vi "WSVCAP SHL FPGA LL Procedure I2C - Read ACK.vi"(0 "Procedure Step":T1, 1 "Wait Ticks Remaining":u32, 7 "I2C Wait Ticks":u32, 9 "Socket Mask":u64 format="%012x", 11 "error in (no error)":errorcluster, 14 "UUT Set (0/1)":u8) -> (3 "Wait Ticks Remaining Out":u32, 4 "Procedure Step Out":T1, 8 "Finished":bool, 10 "ACK Bit Read":u64, 15 "error out":errorcluster)   [LabVIEW 2017]
uses:
  Type Defs/WSVCAP SHL Procedure Step Enum.ctl
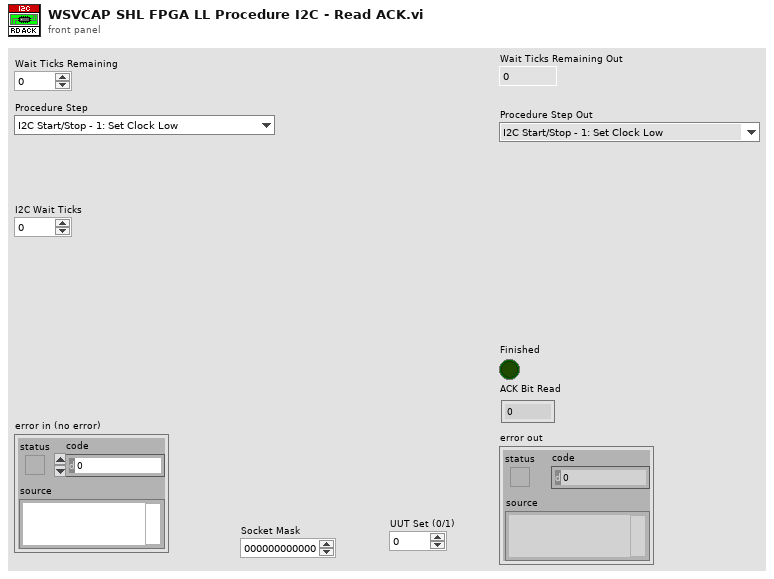
[diagram p1: front panel]
types:
  T1 = typedef "WSVCAP SHL Procedure Step Enum.ctl" = enum16{"I2C Start/Stop - 1: Set Clock Low", "I2C Start/Stop - 2: Wait", "I2C Start/Stop - 3: Set Data I", "I2C Start/Stop - 4: Wait", "I2C Start/Stop - 5: Set Clock High", "I2C Start/Stop - 6: Wait", "I2C Start/Stop - 7: Set Data II", "I2C Start/Stop - 8: Wait", "I2C Start/Stop - 9: Set Clock Low", "I2C Start/Stop - 10: Wait", "I2C Read ACK - 1: Set Clock High", "I2C Read ACK - 2: Wait", "I2C Read ACK - 3: Read ACK Bit", "I2C Read ACK - 4: Wait", "I2C Read ACK - 5: Set Clock Low", "I2C Read ACK - 6: Wait", "I2C Write ACK - 1: Write ACK Bit", "I2C Write ACK - 2: Wait", "I2C Write ACK - 3: Set Clock High", "I2C Write ACK - 4: Wait", "I2C Write ACK - 5: Set Clock Low", "I2C Write ACK - 6: Wait", "I2C Write ACK - 7: Set Data Low", "I2C Send Add - 1: Reset Bits Remaining", "I2C Send Add - 2: Set Data Bit", "I2C Send Add - 3: Wait", "I2C Send Add - 4: Set Clock High", "I2C Send Add - 5: Wait", "I2C Send Add - 6: Set Clock Low", "I2C Send Add - 7: Wait", "I2C Send Add - 8: Check Bits Remaining", "I2C Send Data - 1: Reset Bits Remaining", "I2C Send Data - 2: Load Write Bit from FIFO", "I2C Send Data - 3: Set Data Bit", "I2C Send Data - 4: Wait", "I2C Send Data - 5: Set Clock High", "I2C Send Data - 6: Wait", "I2C Send Data - 7: Set Clock Low", "I2C Send Data - 8: Wait", "I2C Send Data - 9: Check Bits Remaining", "I2C Receive Data - 1: Reset Bits Remaining", "I2C Receive Data - 2: Wait", "I2C Receive Data - 3: Set Clock High", "I2C Receive Data - 4: Wait", "I2C Receive Data - 5: Read Data Bit", "I2C Receive Data - 6: Wait", "I2C Receive Data - 7: Set Clock Low", "I2C Receive Data - 8: Wait", "I2C Receive Data - 9: Check Bits Remaining", "RFFE Send SSC - 1:Set Low", "RFFE Send SSC - 2:Wait", "RFFE Send SSC - 3:Set SDA High", "RFFE Send SSC - 4:Wait", "RFFE Send SSC - 5:Set SDA Low", "RFFE Send SSC - 6:Wait", "RFFE Send Data - 1:Set SCL High", "RFFE Send Data - 2:Wait", "RFFE Send Data - 3:Set SCL Low", "RFFE Send Data - 4:Wait", "RFFE Send Data - 5:Set SCL High (P)", "RFFE Send Data - 6:Wait", "RFFE Send Data - 7:Set SCL Low (P)", "RFFE Send Data - 8:Wait", "RFFE Send Data - 9:Set SCL High (BP)", "RFFE Send Data - 10:Wait", "RFFE Send Data - 11:Set SCL Low (BP)", "RFFE Send Data - 12:Wait", "RFFE Receive Data - 1:Set SCL High", "RFFE Receive Data - 2:Wait", "RFFE Receive Data - 3:Set SCL Low", "RFFE Receive Data - 4:Wait", "RFFE Receive Data - 5:Set SCL High (BP)", "RFFE Receive Data - 6:Wait", "RFFE Receive Data - 7:Set SCL Low (BP)", "RFFE Receive Data - 8:Wait", "RFFE Wait CMD Delay - 1:Wait", "RFFE Clear Lines - 1:Clear"}
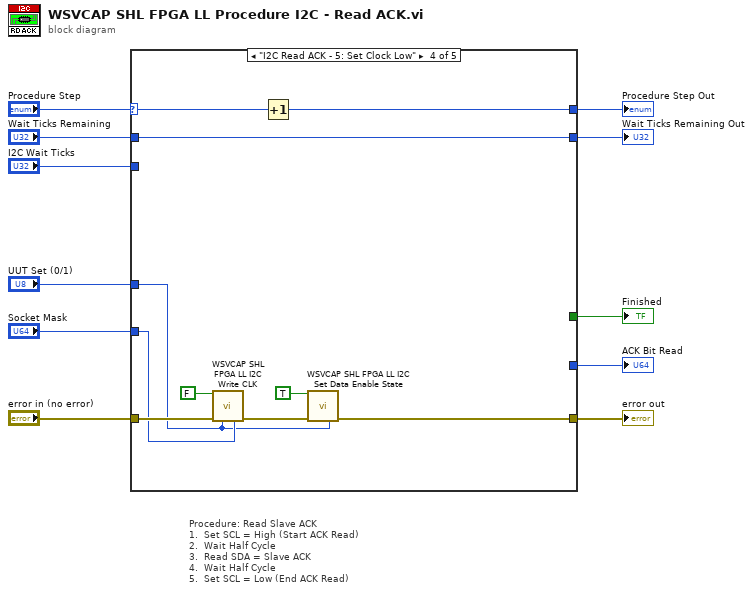
[diagram p0: block diagram]
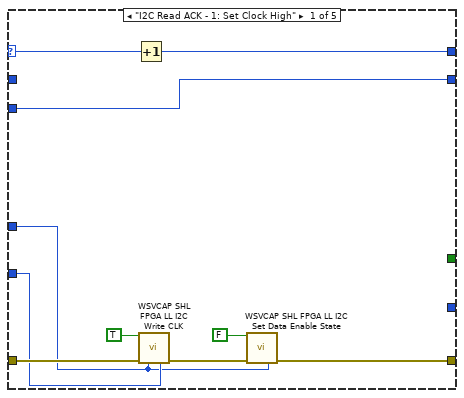
[diagram p2: hidden frame]
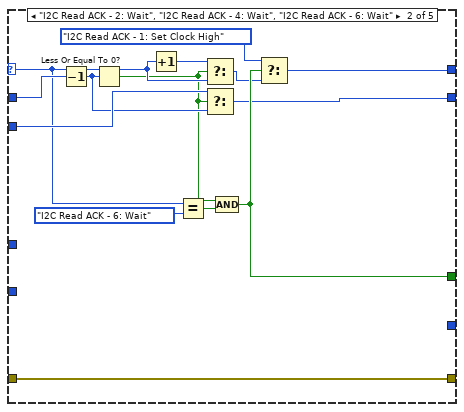
[diagram p3: hidden frame]
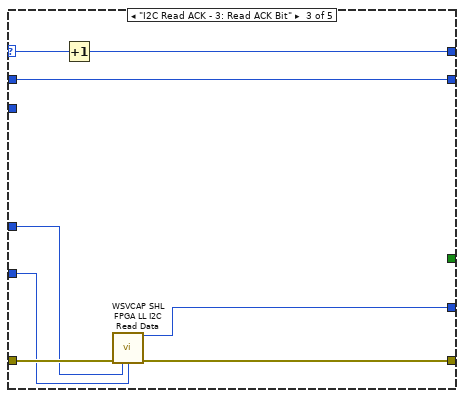
[diagram p4: hidden frame]
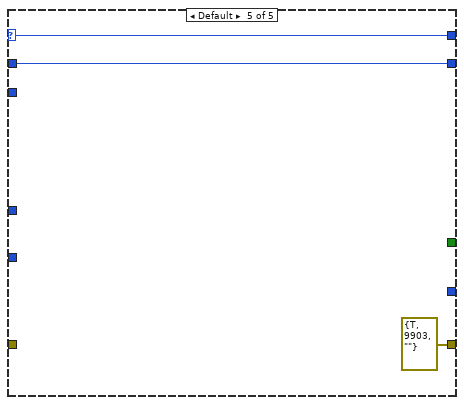
[diagram p5: hidden frame]
diagram:
  # "Procedure: Read Slave ACK\n1.  Set SCL = High (Start ACK Read)\n2.  Wait Half Cycle\n3.  Read SDA = Slave ACK\n4.  Wait Half Cycle\n5.  Set SCL = Low (End ACK Read)"
  n1 = case shown="\"I2C Read ACK - 5: Set Clock Low\"" "Procedure Step" {
    selector: "Procedure Step" -> [w19 w30 w41 w48 w55]
    tunnel: [w17 w33 w42 w50 errorcluster {"status"=TRUE, "code"=9903, "source"=""} ("error out")] -> w10
    tunnel: "error in (no error)" -> [w21 w33 w43 w53 _]
    tunnel: "Wait Ticks Remaining" -> [_ w35 w37 w45 w54]
    tunnel: "I2C Wait Ticks" -> [w13 w32 _ _ _]
    tunnel: [_ w27 _ _ _] -> w9
    tunnel: [_ _ w40 _ _] -> w8
    tunnel: "Socket Mask" -> [w15 _ w39 w47 _]
    tunnel: [w13 w23 w37 w45 w54] -> w3
    tunnel: [w14 w22 w38 w46 w55] -> w2
    tunnel: "UUT Set (0/1)" -> [w12 _ w36 w44 _]
    frame "I2C Read ACK - 1: Set Clock High" {
      n2 = Increment(x=w19) -> (x+1=w14:T1)
      n3 = call "WSVCAP SHL FPGA LL I2C Write CLK.vi"("Bit In"=TRUE, "error in (no error)"=w21, "UUT Set (0/1 (Legacy)"=w12, "Socket Mask"=w15) -> ("error out"=w18:errorcluster)  [unwired: 11 in]
      n4 = call "WSVCAP SHL FPGA LL I2C Set Data Enable State.vi"("State"=FALSE, "error in (no error)"=w18, "UUT Set (0/1)"=w12) -> ("error out"=w17:errorcluster)  [unwired: 12 in]
    }
    frame "I2C Read ACK - 2: Wait", "I2C Read ACK - 4: Wait", "I2C Read ACK - 6: Wait" {
      n5 = Decrement(x=w35) -> (x-1=w31:u32)
      n6 = Less Or Equal To 0?(x=w31) -> (x <= 0?=w29:bool)
      n7 = Increment(x=w30) -> (x+1=w34:T1)
      n8 = Equal?(x=w30, y=WSVCAP_SHL_Procedure_Step_Enum."I2C Read ACK - 6: Wait" ("Procedure Step")) -> (x = y?=w28:bool)
      n9 = Select(t=w34, s=w29, f=w30) -> (s? t:f=w26:T1)
      n10 = Select(t=w32, s=w29, f=w31) -> (s? t:f=w23:u32)
      n11 = Compound Arithmetic op=AND(w29, w28) -> (w27:bool)
      n12 = Select(t=WSVCAP_SHL_Procedure_Step_Enum."I2C Read ACK - 1: Set Clock High" ("Procedure Step"), s=w27, f=w26) -> (s? t:f=w22:T1)
    }
    frame "I2C Read ACK - 3: Read ACK Bit" {
      n13 = Increment(x=w41) -> (x+1=w38:T1)
      n14 = call "WSVCAP SHL FPGA LL I2C Read Data.vi"("error in (no error)"=w43, "UUT Set (0-1) (Legacy)"=w36, "Socket Mask"=w39) -> ("Long Word Out (1-Bit for Each Channel)"=w40:u64, "error out"=w42:errorcluster)  [unwired: 11 in]
    }
    frame "I2C Read ACK - 5: Set Clock Low" {
      n15 = call "WSVCAP SHL FPGA LL I2C Write CLK.vi"("Bit In"=FALSE, "error in (no error)"=w53, "UUT Set (0/1 (Legacy)"=w44, "Socket Mask"=w47) -> ("error out"=w51:errorcluster)  [unwired: 11 in]
      n16 = Increment(x=w48) -> (x+1=w46:T1)
      n17 = call "WSVCAP SHL FPGA LL I2C Set Data Enable State.vi"("State"=TRUE, "error in (no error)"=w51, "UUT Set (0/1)"=w44) -> ("error out"=w50:errorcluster)  [unwired: 12 in]
    }
    frame Default {
    }
  }
  "error out" <- w10
  "Finished" <- w9
  "ACK Bit Read" <- w8
  "Wait Ticks Remaining Out" <- w3
  "Procedure Step Out" <- w2
